vi "test.vi"(8 "字符串与值[]":T1, 11 "按键名字":string(combo)) -> ()   [LabVIEW 2019]
uses:
  <vilib>/Utility/miscctls.llb/LVComboBoxStrsAndValuesArrayTypeDef.ctl
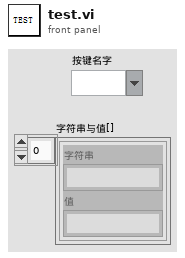
[diagram p1: front panel]
types:
  T1 = typedef "LVComboBoxStrsAndValuesArrayTypeDef.ctl" = cluster{"String":string, "Value":string}[]
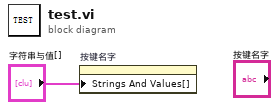
[diagram p0: block diagram]
diagram:
  n1 = property on="按键名字" class="CmbBox"("Strings And Values[]"="字符串与值[]") -> ()  [unwired: 2 in, 2 out]
